vi "DAQ Programming.vi"() -> ()   [LabVIEW 2017]
panel:
  in  "device name":tag="Multifunction"
  out "Thermometer":dbl(slide) scale=0.0..100.0
  out "Current (A)":dbl(knob) scale=0.0..10.0
  out "Voltage (V)":dbl(knob) scale=0.0..10.0
  in  "stop":bool
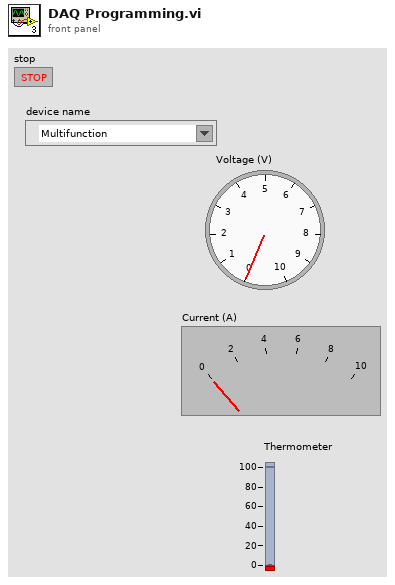
[diagram p1: front panel]
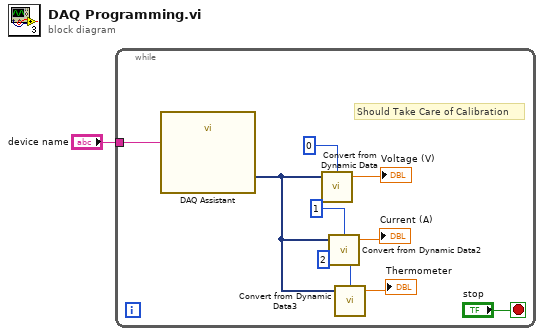
[diagram p0: block diagram]
diagram:
  n1 = while {
    tunnel: "device name" -> [w2]
    stop <- "stop" stop-if-true
    # "Should Take Care of Calibration"
    n2 = call "DAQ Assistant"("device name"=w2) -> ("data"=w6:dynamicdata)  [unwired: 16 in, 2 out]
    n3 = call "Convert from Dynamic Data"("Dynamic Data Type"=w6, "Channel"=0) -> ("Scalar"=→"Voltage (V)":dbl)  [unwired: 2 in]
    n4 = call "Convert from Dynamic Data2"("Dynamic Data Type"=w6, "Channel"=1) -> ("Scalar"=→"Current (A)":dbl)  [unwired: 2 in]
    n5 = call "Convert from Dynamic Data3"("Dynamic Data Type"=w6, "Channel"=2) -> ("Scalar"=→"Thermometer":dbl)  [unwired: 2 in]
  }
